vi "get_default_voltage.vi"(8 "error in (no error)":errorcluster, 11 "DAQmxAnalogOut.lvclass in":refnum<class "AnalogOutDL101207DAQmx.lvclass">) -> (0 "error out":errorcluster, 2 "default voltage":dbl[unit], 3 "DAQmxAnalogOut.lvclass out":refnum<class "AnalogOutDL101207DAQmx.lvclass">)   [LabVIEW 2010, in "AnalogOutDL101207DAQmx.lvclass"]
uses:
  AnalogOutDL101207DAQmx.lvclass
  AnalogOutDL101207DAQmx.lvclass/AnalogOutDL101207DAQmx.ctl
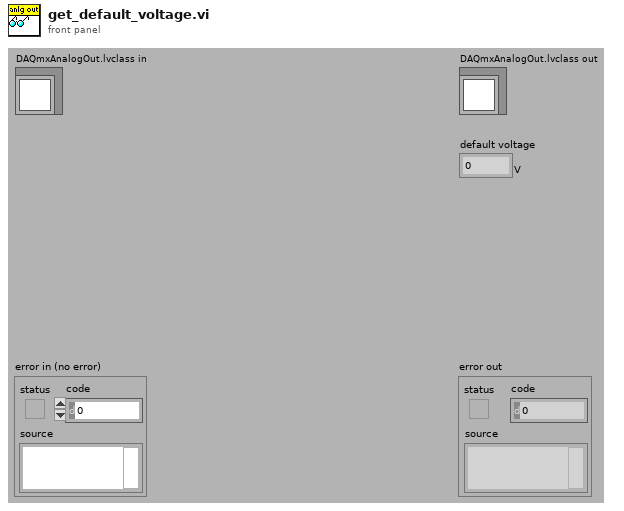
[diagram p1: front panel]
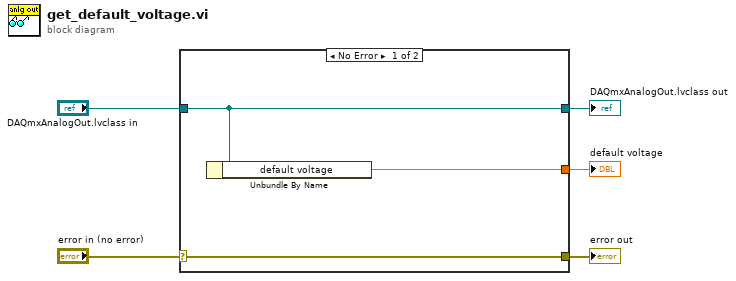
[diagram p0: block diagram]
diagram:
  n1 = case shown="No Error" "error in (no error)" {
    selector: "error in (no error)" -> [w8 w9]
    tunnel: [w8 w9] -> w4
    tunnel: [w7 w10] -> w2
    tunnel: "DAQmxAnalogOut.lvclass in" -> [w7 w10]
    tunnel: [w6 _] -> w1
    frame No Error {
      n2 = Unbundle By Name(w7) -> ("default voltage"=w6:dbl[unit])
    }
    frame Error {
    }
  }
  "error out" <- w4
  "DAQmxAnalogOut.lvclass out" <- w2
  "default voltage" <- w1
